vi "StartSequence.vi"(8 "error in (no error)":errorcluster, 9 "SeqLength":i32, 11 "ExecutionStatus in":refnum<class "ExecutionStatus.lvclass">) -> (0 "error out":errorcluster, 3 "ExecutionStatus out":refnum<class "ExecutionStatus.lvclass">)   [LabVIEW 2019, in "ExecutionStatus.lvclass"]
uses:
  ExecutionStatus.lvclass
  ExecutionStatus.lvclass/ExecutionStatus.ctl
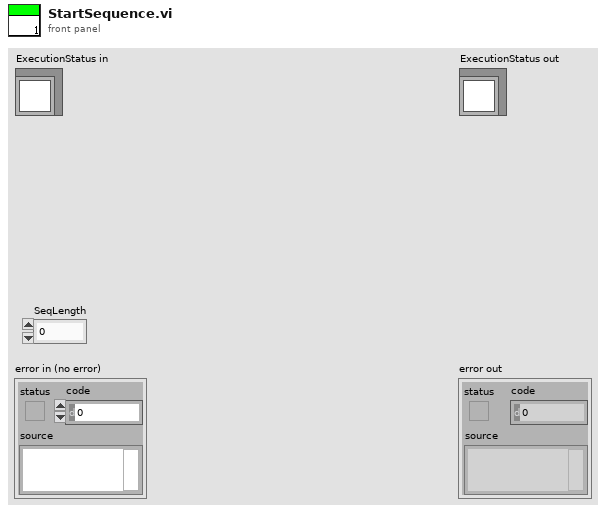
[diagram p1: front panel]
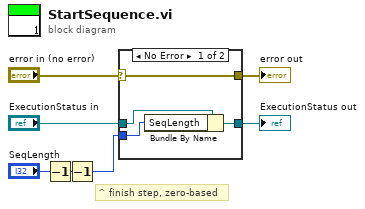
[diagram p0: block diagram]
diagram:
  # "^ finish step, zero-based"
  n1 = Decrement(x="SeqLength") -> (x-1=w1:i32)
  n2 = Decrement(x=w1) -> (x-1=w2:i32)
  n3 = case shown="No Error" "error in (no error)" {
    selector: "error in (no error)" -> [w11 w13]
    tunnel: [w11 w13] -> w6
    tunnel: [w9 w12] -> w4
    tunnel: "ExecutionStatus in" -> [w10 w12]
    tunnel: w2 -> [w8 _]
    frame No Error {
      n4 = Bundle By Name(cluster=w10, "SeqLength"=w8) -> (w9:refnum<class "ExecutionStatus.lvclass">)
    }
    frame Error {
    }
  }
  "error out" <- w6
  "ExecutionStatus out" <- w4
